vi "Program_Device.vi"(8 "error in (no error)":errorcluster, 10 "Parameters":string, 11 "reference in":refnum<class "Test_Flux_Capacitor.lvclass">) -> (0 "error out":errorcluster, 2 "Result":bool, 3 "reference out":refnum<class "Test_Flux_Capacitor.lvclass">)   [LabVIEW 2022 SP3, in "Test_Flux_Capacitor.lvlib" / "Test_Flux_Capacitor.lvclass"]
uses:
  Test_Flux_Capacitor.lvclass
  Components/JTAG_Base.lvlibp/JTAG_Base.lvclass
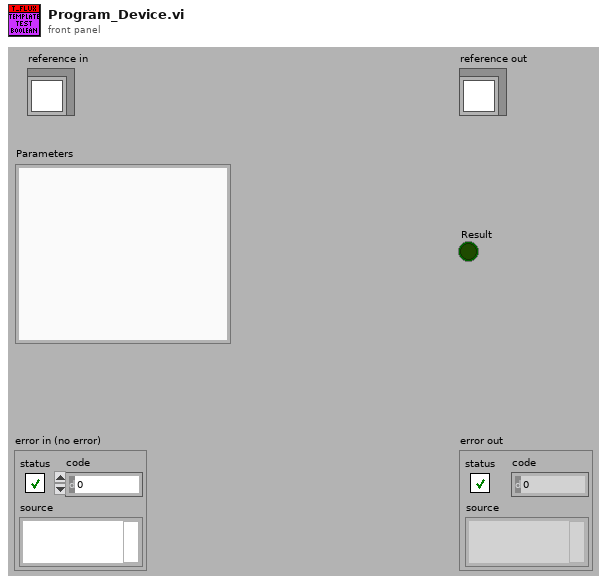
[diagram p1: front panel]
types:
  T1 = typedef "Test_Flux_Capacitor.lvlib/Test_Flux_Capacitor.lvclass/ObjectAttributes.ctl" = cluster{"Config":T2, "DMM":refnum<class "DMM_Keysight_34980A.lvclass">, "LCR":refnum<class "LCR_BK891.lvclass">, "PSU":refnum<class "PSU_Base.lvclass">, "Switch_Manager":refnum<class "SwitchBase.lvclass">, "FRAM":string, "Flux_Capacitor":refnum<class "Flux_Capacitor.lvclass">, "Frequency_Counter":refnum<class "Frequency_Counter_Base.lvclass">, "JTAG":refnum<class "JTAG_Base.lvclass">}
  T2 = typedef "Test_Flux_Capacitor.lvlib/Test_Flux_Capacitor.lvclass/Config.ctl" = cluster{"default":string}
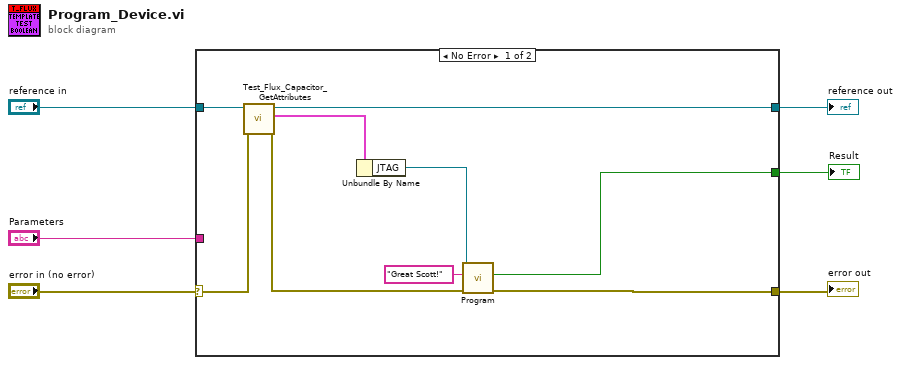
[diagram p0: block diagram]
diagram:
  n1 = case shown="No Error" "error in (no error)" {
    selector: "error in (no error)" -> [w15 w17]
    tunnel: [w9 w17] -> w5
    tunnel: [w13 w16] -> w3
    tunnel: "reference in" -> [w14 w16]
    tunnel: "Parameters" -> [_ _]
    tunnel: [w7 _] -> w1
    frame No Error {
      n2 = call "Test_Flux_Capacitor_GetAttributes.vi"("error in (no error)"=w15, "reference in"=w14) -> ("error out"=w10:errorcluster, "Data"=w12:T1, "reference out"=w13:refnum<class "Test_Flux_Capacitor.lvclass">)  [unwired: 6 in, 1 out]
      n3 = Unbundle By Name(w12) -> ("JTAG"=w11:refnum<class "JTAG_Base.lvclass">)
      n4 = call-dynamic "Program.vi"("error in (no error)"=w10, "Image"="Great Scott!", "reference in"=w11) -> ("error out"=w9:errorcluster, "Success"=w7:bool)  [unwired: 5 in, 2 out]
    }
    frame Error {
    }
  }
  "Result" <- w1
  "error out" <- w5
  "reference out" <- w3
